vi "Measurement Logic.vi"(8 "error in":errorcluster, 9 "measurement configuration":T2={"TREE"="Lorem ipsum dolor sit", "CONNECTIONS"=1, "START"=TRUE, "OPEN SESSION"=FALSE, "OPERATION"=32, "SWITCH EXECUTIVE VIRTUAL DEVICE"="Empty"} {"OPERATION" items=["CONNECT", "DISCONNECT", "DISCONNECT ALL"]}, 10 "measure call context in":refnum<class "Measure Call Context.lvclass">) -> (0 "error out":errorcluster, 1 "measurement results":T1={"START"=FALSE, "OPEN SESSION"=FALSE, "SWITCH EXECUTIVE VIRTUAL DEVICE"="Empty", "TREE"="", "CONNECTIONS"=0, "OPERATION"=0} {"OPERATION" items=["CONNECT", "DISCONNECT", "DISCONNECT ALL"]}, 2 "measure call context out":refnum<class "Measure Call Context.lvclass">)   [LabVIEW 2025, in "NI Switch Control.lvclass"]
doc: "Contains the core logic for executing the measurement."
uses:
  NI Switch Control.lvclass
  <vilib>/Plug-In SDKs/Measurements/Measure Call Context/Measure Call Context.lvclass
  Measurement Configuration.ctl
  Measurement Results.ctl
  <extravilib>/ChannelInstances/Event Messenger-bool/Instantiate.vi
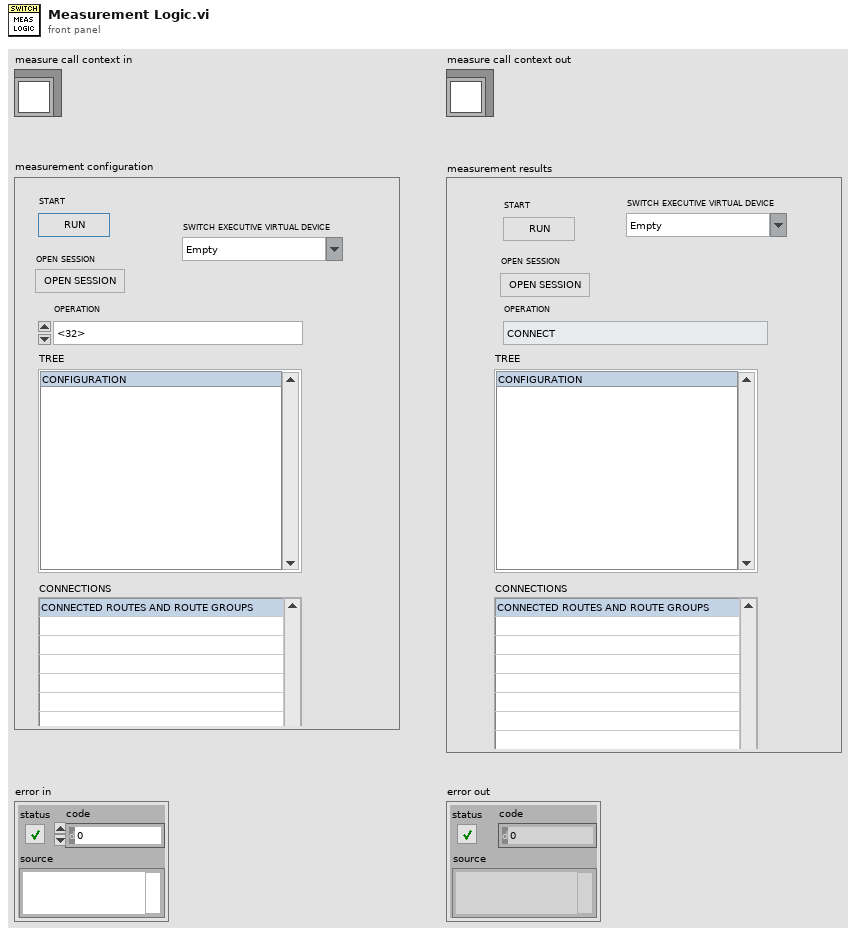
[diagram p1: front panel]
types:
  T1 = typedef "NI Switch Control.lvclass/Measurement Results.ctl" = cluster{"START":bool, "OPEN SESSION":bool, "SWITCH EXECUTIVE VIRTUAL DEVICE":string, "TREE":string, "CONNECTIONS":i32, "OPERATION":i32}
  T2 = typedef "NI Switch Control.lvclass/Measurement Configuration.ctl" = cluster{"TREE":string, "CONNECTIONS":i32, "START":bool, "OPEN SESSION":bool, "OPERATION":i32, "SWITCH EXECUTIVE VIRTUAL DEVICE":string}
  T3 = typedef "Event Messenger-bool.lvlib/))Channel.ctl" = refnum<queue>
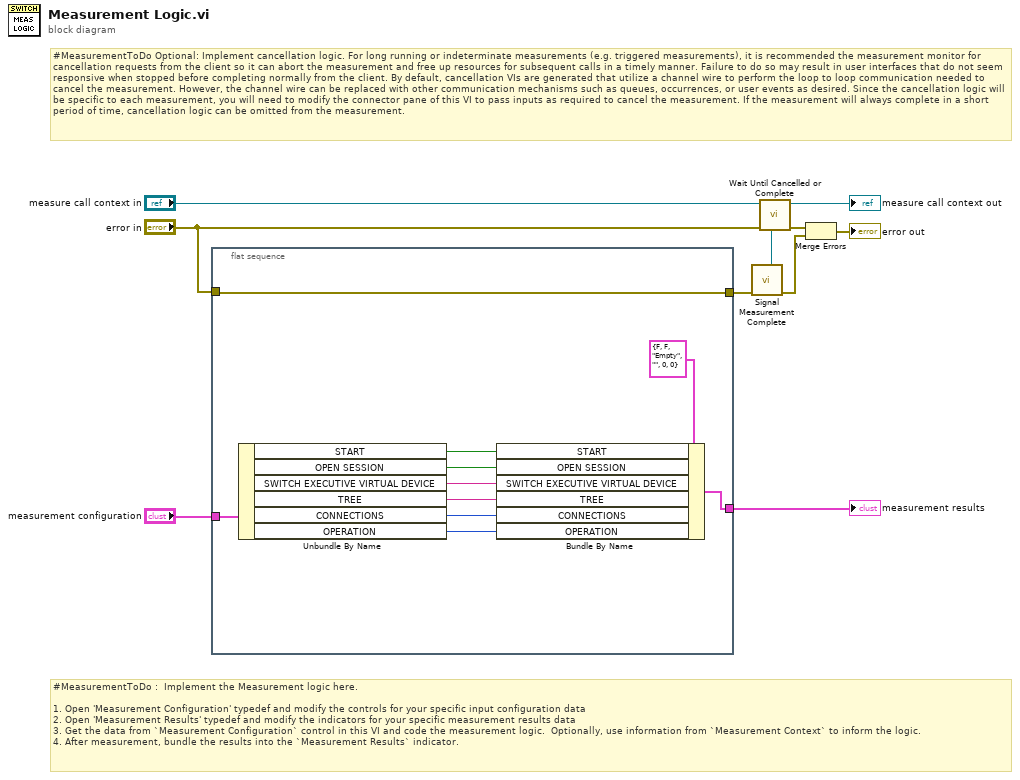
[diagram p0: block diagram]
diagram:
  # "#MeasurementToDo Optional: Implement cancellation logic. For long running or indeterminate measurements (e.g. triggered measurements), it is recommended the measurement monitor for cancellation requests from the client so it can abort the measurement and free up resources for subsequent calls in a timely manner. Failure to do so may result in user interfaces that do not seem responsive when stopped before completing normally from the client. By default, cancellation VIs are generated that utilize a channel wire to perform the loop to loop communication needed to cancel the measurement. However, the channel wire can be replaced with other communication mechanisms such as queues, occurrences, or user events as desired. Since the cancellation logic will be specific to each measurement, you will need to modify the connector pane of this VI to pass inputs as required to cancel the measurement. If the measurement will always complete in a short period of time, cancellation logic can be omitted from the measurement."
  # "#MeasurementToDo :  Implement the Measurement logic here.\n\n1. Open 'Measurement Configuration' typedef and modify the controls for your specific input configuration data\n2. Open 'Measurement Results' typedef and modify the indicators for your specific measurement results data\n3. Get the data from `Measurement Configuration` control in this VI and code the measurement logic.  Optionally, use information from `Measurement Context` to inform the logic.\n4. After measurement, bundle the results into the `Measurement Results` indicator."
  n1 = flat-sequence {
    tunnel: "measurement configuration" -> [w19]
    tunnel: [w17] -> w9
    tunnel: "error in" -> [w20]
    tunnel: [w20] -> w5
    frame #0 {
      n2 = Unbundle By Name(w19) -> ("START"=w16:bool, "OPEN SESSION"=w15:bool, "SWITCH EXECUTIVE VIRTUAL DEVICE"=w14:string, "TREE"=w13:string, "CONNECTIONS"=w12:i32, "OPERATION"=w11:i32)
      n3 = Bundle By Name(cluster=T1 {"START"=FALSE, "OPEN SESSION"=FALSE, "SWITCH EXECUTIVE VIRTUAL DEVICE"="Empty", "TREE"="", "CONNECTIONS"=0, "OPERATION"=0} ("Measurement Results"), "START"=w16, "OPEN SESSION"=w15, "SWITCH EXECUTIVE VIRTUAL DEVICE"=w14, "TREE"=w13, "CONNECTIONS"=w12, "OPERATION"=w11) -> (w17:T1)
    }
  }
  n4 = call "Signal Measurement Complete.vi"("error in (no error)"=w5) -> ("error out"=w3:errorcluster, "done channel"=w4:T3)  [unwired: 9 in]
  n5 = call "Wait Until Cancelled or Complete.vi"("done channel"=w4, "error in (no error)"="error in", "measure call context in"="measure call context in") -> ("error out"=w2:errorcluster, "measure call context out"=→"measure call context out":refnum<class "Measure Call Context.lvclass">)  [unwired: 7 in]
  n6 = Merge Errors(w2, w3) -> (→"error out":errorcluster)
  "measurement results" <- w9
